vi "Determine Analog Outputs from Simple Controls.vi"   [LabVIEW 2010]
uses:
  Motor Output Global.vi
  Motor Encoder Global.vi
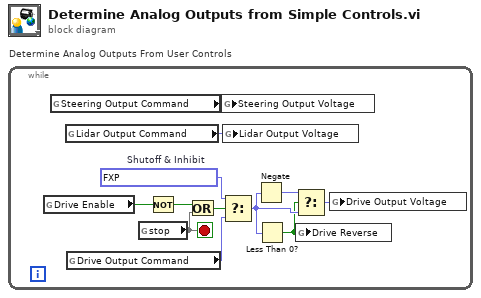
[diagram p0: block diagram]
diagram:
  n1 = while "Determine Analog Outputs From User Controls" {
    stop <- w6 stop-if-true
    w12 = fxp<+/-,20,5> 0.0  # Shutoff & Inhibit
    n2 = global read "Motor Output Global.vi" "Drive Enable"() -> (w7:bool)
    n3 = global read "Motor Output Global.vi" "Steering Output Command"() -> (w2:fxp<+/-,20,5>)
    n4 = global read "Motor Output Global.vi" "Lidar Output Command"() -> (w3:fxp<+/-,20,5>)
    n5 = global read "Motor Output Global.vi" "Drive Output Command"() -> (w1:fxp<+/-,20,5>)
    n6 = global read "Motor Encoder Global.vi" "stop"() -> (w6)
    n7 = Not(x=w7) -> (.not. x?=w11:bool)
    n8 = Or(x=w11, y=w6) -> (x .or. y?=w10:bool)
    n9 = global write "Motor Output Global.vi" "Steering Output Voltage"(w2) -> ()
    n10 = global write "Motor Output Global.vi" "Lidar Output Voltage"(w3) -> ()
    n11 = Select(t=w12, s=w10, f=w1) -> (s? t:f=w9:fxp<+/-,20,5>)
    n12 = Negate(x=w9) -> (-x=w8:fxp<+/-,20,5>)
    n13 = Less Than 0?(x=w9) -> (x < 0?=w4:bool)
    n14 = Select(t=w8, s=w4, f=w9) -> (s? t:f=w5:fxp<+/-,20,5>)
    n15 = global write "Motor Output Global.vi" "Drive Reverse"(w4) -> ()
    n16 = global write "Motor Output Global.vi" "Drive Output Voltage"(w5) -> ()
  }
